vi "Oculus Rift Controller.vi"   [LabVIEW 2014, in "Controller Library.lvlib" / "Oculus Rift Controller.lvclass"]
uses:
  Oculus Rift Controller.lvclass
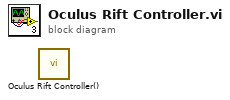
[diagram p0: block diagram]
diagram:
  n1 = call "Oculus Rift Controller().vi"() -> ()  [unwired: 11 in, 1 out]
